vi "VariantArrayAccess1D.vi"(8 "error in (no error)":errorcluster, 10 "index":i32, 11 "Array":variant) -> (0 "error out":errorcluster, 1 "rest":string, 2 "value":variant, 3 "prepend":string, 5 "array size":u32[](array[numeric]), 7 "type string":i16[](array[numeric]))   [LabVIEW 2020]
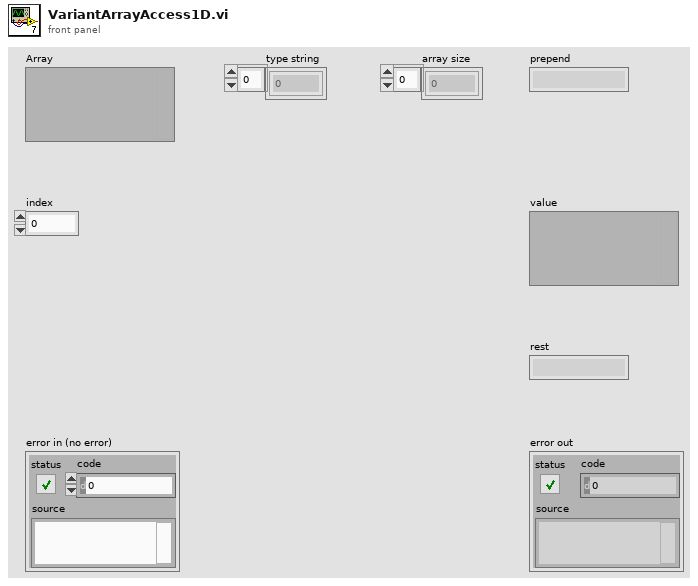
[diagram p1: front panel]
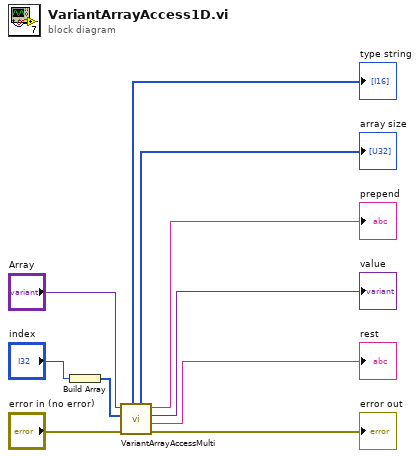
[diagram p0: block diagram]
diagram:
  n1 = Build Array("index") -> (w10:i32[])
  n2 = call "VariantArrayAccessMulti.vi"("error in (no error)"="error in (no error)", "Indices"=w10, "Array"="Array") -> ("error out"=→"error out":errorcluster, "rest"=→"rest":string, "value"=→"value":variant, "prepend"=→"prepend":string, "array size"=→"array size":u32[], "type string"=→"type string":i16[])  [unwired: 3 in]
